vi "InitDone.vi"(8 "error in (no error)":errorcluster, 9 "instr error":errorcluster, 10 "Address":T1, 11 "InterferometrUI in":refnum<class "InterferometerUI.lvclass">) -> (0 "error out":errorcluster, 3 "InterferometrUI out":refnum<class "InterferometerUI.lvclass">)   [LabVIEW 2023, in "InterferometrUI.lvlib" / "InterferometerUI.lvclass"]
uses:
  InterferometerUI.lvclass
  InterferometerUI.lvclass/InterferometerUI.ctl
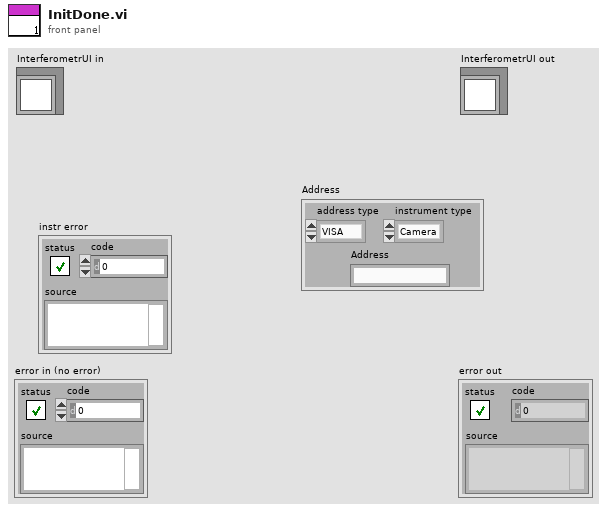
[diagram p1: front panel]
types:
  T1 = cluster{"address type":enum16{"VISA", "Index"}, "Address":string, "instrument type":enum16{"Camera", "Stepper"}}
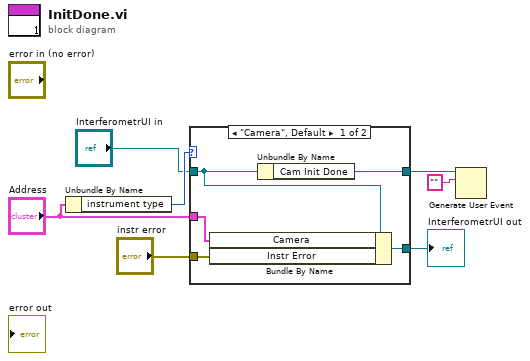
[diagram p0: block diagram]
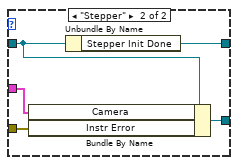
[diagram p2: hidden frame]
diagram:
  n1 = Unbundle By Name("Address") -> ("instrument type"=w6:enum16{"Camera", "Stepper"})
  n2 = case shown="\"Camera\", Default" w6 {
    tunnel: "InterferometrUI in" -> [w11 w14]
    tunnel: [w12 w17] -> w4
    tunnel: [w10 w13] -> w3
    tunnel: "Address" -> [w8 w16]
    tunnel: "instr error" -> [w9 w15]
    frame "Camera", Default {
      n3 = Bundle By Name(cluster=w11, "Camera"=w8, "Instr Error"=w9) -> (w10:refnum<class "InterferometerUI.lvclass">)
      n4 = Unbundle By Name(w11) -> ("Cam Init Done"=w12:refnum<user-event>)
    }
    frame "Stepper" {
      n5 = Bundle By Name(cluster=w14, "Camera"=w16, "Instr Error"=w15) -> (w13:refnum<class "InterferometerUI.lvclass">)
      n6 = Unbundle By Name(w14) -> ("Stepper Init Done"=w17:refnum<user-event>)
    }
  }
  "InterferometrUI out" <- w3
  n7 = Generate User Event(user event=w4, event data cluster="" ("event data")) -> ()  [unwired: 2 in, 2 out]
